vi "Write Timeout.vi"(8 "error in (no error)":errorcluster, 10 "Timeout":i32=10000, 11 "REST Client in":refnum<class "REST Client.lvclass">) -> (0 "error out":errorcluster, 3 "REST Client out":refnum<class "REST Client.lvclass">)   [LabVIEW 2013, in "REST Client.lvlib" / "REST Client.lvclass"]
uses:
  REST Client.lvclass
  REST Client.lvclass/REST Client.ctl
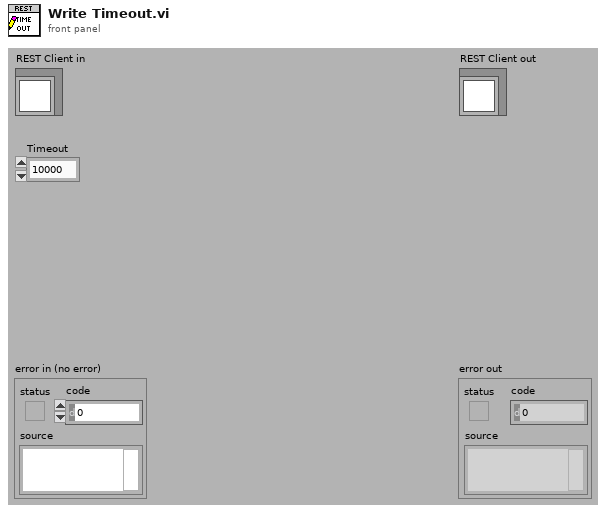
[diagram p1: front panel]
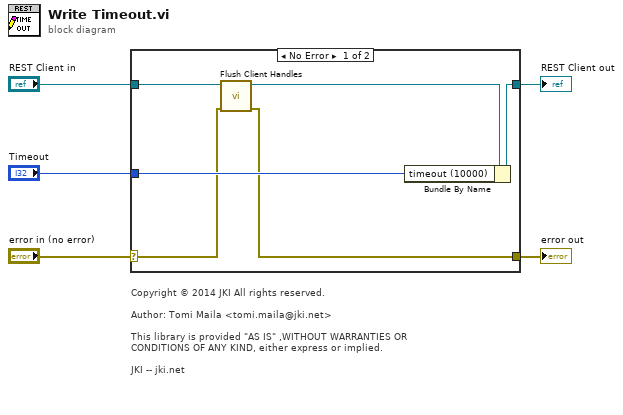
[diagram p0: block diagram]
diagram:
  # "Copyright © 2014 JKI All rights reserved.\n\nAuthor: Tomi Maila <tomi.maila@jki.net>\n\nThis library is provided \"AS IS\" ,WITHOUT WARRANTIES OR \nCONDITIONS OF ANY KIND, either express or implied.\n\nJKI -- jki.net"
  n1 = case shown="No Error" "error in (no error)" {
    selector: "error in (no error)" -> [w7 w12]
    tunnel: [w6 w12] -> w4
    tunnel: [w11 w13] -> w2
    tunnel: "REST Client in" -> [w9 w13]
    tunnel: "Timeout" -> [w10 _]
    frame No Error {
      n2 = call-dynamic "Flush Client Handles.vi"("error in (no error)"=w7, "REST Client in"=w9) -> ("error out"=w6:errorcluster, "REST Client out"=w8:refnum<class "REST Client.lvclass">)  [unwired: 8 in]
      n3 = Bundle By Name(cluster=w8, "timeout (10000)"=w10) -> (w11:refnum<class "REST Client.lvclass">)
    }
    frame Error {
    }
  }
  "error out" <- w4
  "REST Client out" <- w2
